vi "Aux Device (Set).vi"(6 "ISOBUS address":T5=-1 caption="ISOBUS address (-1)", 8 "error in":errorcluster, 10 "Auxiliary Device":T3 {"Signals"."% Open" min=0.0 max=100.0 step=0.1 format="%#.1f"; "Speed" max=7 step=1; "Gear" max=7 step=1; "Temp V Err" min=0.0 max=20.0 step=0.1; "Temp Err" min=0.0 max=20.0 step=0.1; "Scaling Factor" min=0.0 max=99.0 step=0.1; "Min Flow" min=0.0 max=20.0 step=0.1}, 11 "Mercury Reference In":T6) -> (0 "error out":errorcluster, 2 "Response":T1, 3 "Mercury Reference Out":T6, 4 "Valid?":T2)   [LabVIEW 2015, in "Mercury iXX.lvlib" / "Auxiliary.lvlib"]
doc: "Set the auxiliary device configuration."
uses:
  Auxiliary.lvlib
  Controls/Mercury Reference.ctl
  Controls/Comms Transport Layer.ctl
  private/Controls/Query Dynamic Reference.ctl
  Controls/ISOBus Address.ctl
  Controls/AUX Device (Set).ctl
  Controls/AUX Signals (Set).ctl
  Controls/Is Valid LED.ctl
  Controls/Response String.ctl
  private/Controls/Command Verbs.ctl
  Mercury iXX.lvlib
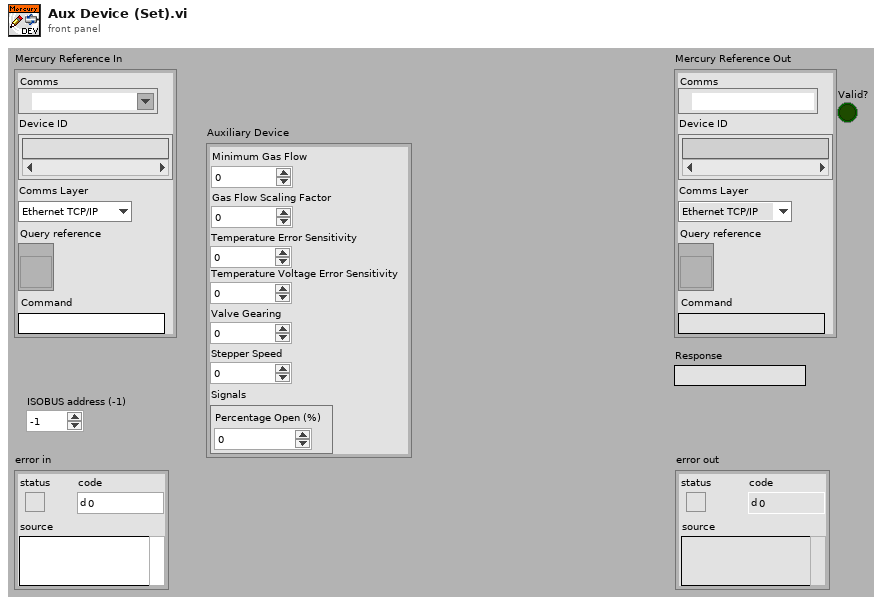
[diagram p1: front panel]
types:
  T1 = typedef "Mercury iXX.lvlib/Response String.ctl" = string
  T2 = typedef "Mercury iXX.lvlib/Is Valid LED.ctl" = bool
  T3 = typedef "Mercury iXX.lvlib/Auxiliary.lvlib/AUX Device (Set).ctl" = cluster{"Min Flow":dbl, "Scaling Factor":dbl, "Temp Err":dbl, "Temp V Err":dbl, "Gear":u32, "Speed":u32, "Signals":T4}
  T4 = typedef "Mercury iXX.lvlib/Auxiliary.lvlib/AUX Signals (Set).ctl" = cluster{"% Open":dbl}
  T5 = typedef "Mercury iXX.lvlib/ISOBus Address.ctl" = i32
  T6 = typedef "Mercury iXX.lvlib/Mercury Reference.ctl" = cluster{"Comms":refnum<visa-resource-name>, "Device ID":string[], "Comms Layer":T7, "Command":string, "Query reference":T8}
  T7 = typedef "Mercury iXX.lvlib/Comms Transport Layer.ctl" = enum16{"Ethernet TCP/IP", "USB", "ISOBus - RS-232", "GPIB"}
  T8 = typedef "Mercury iXX.lvlib/Query Dynamic Reference.ctl" = refnum<vi>
  T9 = typedef "Mercury iXX.lvlib/Command Verbs.ctl" = string
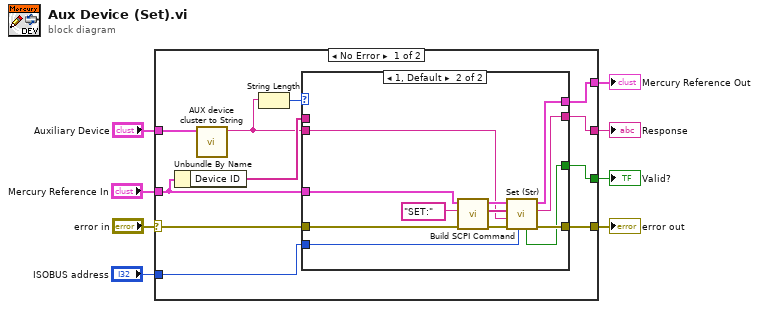
[diagram p0: block diagram]
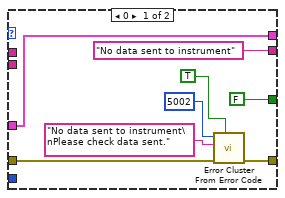
[diagram p2: hidden frame]
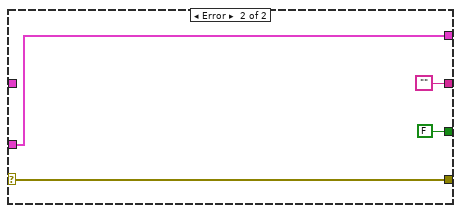
[diagram p3: hidden frame]
diagram:
  n1 = case shown="No Error" "error in" {
    selector: "error in" -> [w19 w42]
    tunnel: "Mercury Reference In" -> [w14 w43]
    tunnel: [w15 w43] -> w7
    tunnel: [w16 w42] -> w6
    tunnel: "ISOBUS address" -> [w18 _]
    tunnel: [w10 ""] -> w2
    tunnel: [w9 FALSE ("Valid?")] -> w3
    tunnel: "Auxiliary Device" -> [w12 _]
    frame No Error {
      n2 = Unbundle By Name(w14) -> ("Device ID"=w17:string[])
      n3 = call "AUX device cluster to String.vi"("Auxiliary Device"=w12) -> ("Data to send"=w11:string)  [unwired: 10 out]
      n4 = String Length(string=w11) -> (length=w13:i32)
      n5 = case shown="1, Default" w13 {
        tunnel: ["No data sent to instrument" ("Data") w30] -> w10
        tunnel: [FALSE ("Valid?") w28] -> w9
        tunnel: w14 -> [w27 w35]
        tunnel: w17 -> [_ _]
        tunnel: w18 -> [_ w32]
        tunnel: w19 -> [w25 w33]
        tunnel: [w26 w31] -> w16
        tunnel: [w27 w29] -> w15
        tunnel: w11 -> [_ w34]
        frame 0 {
          n6 = call <vilib>:"Error Cluster From Error Code.vi"("show call chain? (False)"=TRUE, "error in (no error)"=w25, "error message (\"\")"="No data sent to instrument\nPlease check data sent." ("error message (\"\")"), "error code (0)"=5002) -> ("error out"=w26:errorcluster)  [unwired: 5 out]
        }
        frame 1, Default {
          n7 = call "Build SCPI Command.vi"("error in"=w33, "Verb"=T9 "SET:", "Mercury Reference In"=w35) -> ("error out"=w37:errorcluster, "SCPI Message(s)"=w38:string[], "Mercury Reference Out"=w39:T6)  [unwired: 1 in, 5 out]
          n8 = call "Set (Str).vi"("ISOBUS address"=w32, "error in"=w37, "Command Value (Str)"=w34, "SCPI Message(s)"=w38, "Mercury Reference In"=w39) -> ("error out"=w31:errorcluster, "Response"=w30:T1, "Mercury Reference Out"=w29:T6, "Valid?"=w28:T2)  [unwired: 3 out]
        }
      }
    }
    frame Error {
    }
  }
  "Mercury Reference Out" <- w7
  "error out" <- w6
  "Valid?" <- w3
  "Response" <- w2
